vi "Read Header.vi"(8 "error in (no error)":errorcluster, 11 "Request in":refnum<class "Request.lvclass">) -> (0 "error out":errorcluster, 3 "Request out":refnum<class "Request.lvclass">)   [LabVIEW 2023, in "Request.lvclass"]
doc: "Read the entire header block from the HTTP request."
uses:
  Request.lvclass
  Request.lvclass/Request.ctl
  <vilib>/Utility/error.llb/Trim Whitespace One-Sided.vi
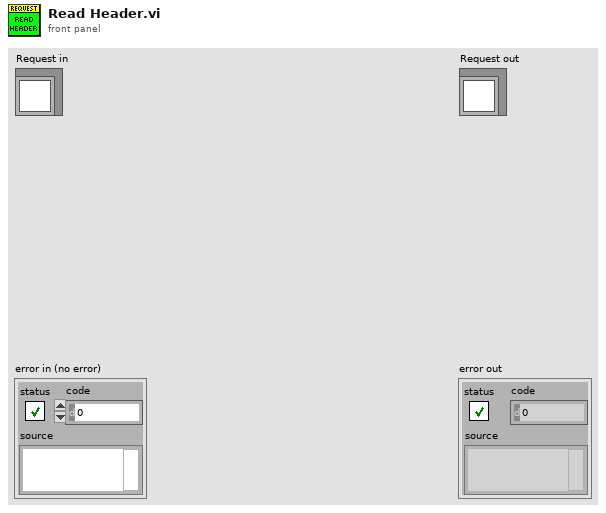
[diagram p1: front panel]
types:
  T1 = enum16{"Standard", "Buffered", "CRLF", "Immediate"}
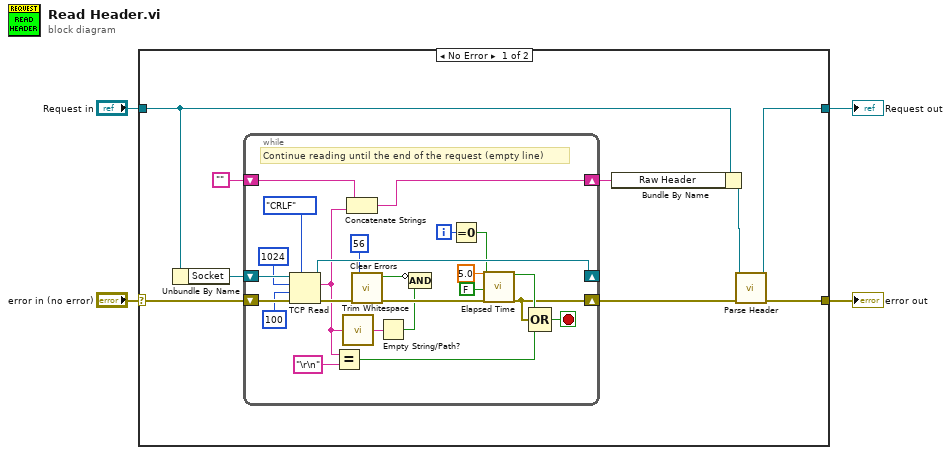
[diagram p0: block diagram]
diagram:
  n1 = case shown="No Error" "error in (no error)" {
    selector: "error in (no error)" -> [w13 w39]
    tunnel: [w7 w39] -> w3
    tunnel: [w5 w38] -> w1
    tunnel: "Request in" -> [w10 w38]
    frame No Error {
      n2 = Unbundle By Name(w10) -> ("Socket"=w12:refnum<k5>)
      n3 = while {
        shift-right: [w32] -> w9
        shift-left: "" -> [w33]
        shift-right: [w30] -> _
        shift-left: w12 -> [w37]
        shift-right: [w14] -> w8
        shift-left: w13 -> [w36]
        i -> [w19]
        stop <- w27 stop-if-true
        # "Continue reading until the end of the request (empty line)"
        n4 = TCP Read(connection ID=w37, bytes to read=1024, error in (no error)=w36, 7:T1."CRLF" ("mode (standard)"), 9:100 ("timeout ms (wait forever: -1)")) -> (connection ID out=w30:refnum<k5>, data out=w22:string, error out=w28:errorcluster)
        n5 = Equal?(x=w22, y="\r\n") -> (x = y?=w20:bool)
        n6 = call <vilib>:"Trim Whitespace.vi"("string"=w22) -> ("trimmed string"=w29:string)  [unwired: 1 in]
        n7 = Concatenate Strings(w33, w22) -> (w32:string)
        n8 = call <vilib>:"Clear Errors.vi"("error in (no error)"=w28, "specific error code to clear (0: all)"=56 ("bytes to read")) -> ("error out"=w26:errorcluster, "specific error cleared?"=w23:bool)  [unwired: 4 in]
        n9 = Empty String/Path?(string/path=w29) -> (empty?=w24:bool)
        n10 = Compound Arithmetic op=AND(invert w23, w24) -> ()  [unwired: 1 out]
        n11 = Equal To 0?(x=w19) -> (x = 0?=w18:bool)
        n12 = call "Elapsed Time.vi"("Reset"=w18, "Elapsed Time Target"=5.0, "Auto Reset"=FALSE, "error in (no error)"=w26) -> ("Time has Elapsed"=w15:bool, "error out"=w14:errorcluster)  [unwired: 10 in, 4 out]
        n13 = Compound Arithmetic op=OR(w15, w14, w20) -> (w27:bool)
      }
      n14 = Bundle By Name(cluster=w10, "Raw Header"=w9) -> (w6:refnum<class "Request.lvclass">)
      n15 = call "Parse Header.vi"("error in (no error)"=w8, "Request in"=w6) -> ("error out"=w7:errorcluster, "Request out"=w5:refnum<class "Request.lvclass">)  [unwired: 8 in]
    }
    frame Error {
    }
  }
  "error out" <- w3
  "Request out" <- w1
